vi "State Helper.vi"(0 "new state":bool, 1 "old state":bool) -> (2 "new state is True?":bool, 3 "new state is False?":bool, 4 "new state changed to True?":bool, 5 "new state changed to False?":bool)   [LabVIEW 2016, in "Hardware.lvlib" / "Motions.lvlib" / "Motions.lvclass"]
uses:
  <userlib>/Common Components/Hardware/Abstract System/Motions/Motions/Motions.lvclass
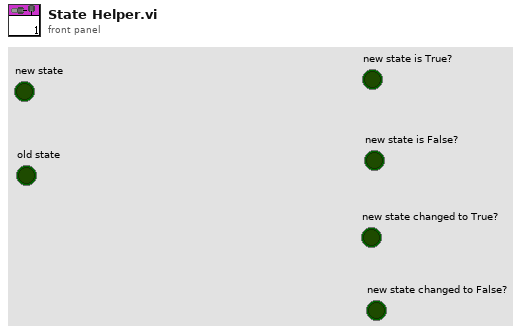
[diagram p1: front panel]
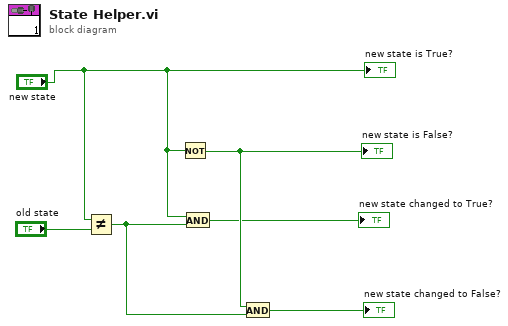
[diagram p0: block diagram]
diagram:
  n1 = Not Equal?(x="new state", y="old state") -> (x != y?=w3:bool)
  n2 = Not(x="new state") -> (.not. x?=w4:bool)
  "new state is False?" <- w4
  n3 = And(x="new state", y=w3) -> (x .and. y?=→"new state changed to True?":bool)
  n4 = And(x=w4, y=w3) -> (x .and. y?=→"new state changed to False?":bool)
  "new state is True?" <- "new state"
